vi "Find Rounded Error.vi"(1 "Camera Angle":dbl=35.25, 2 "Camera Axis Position":dbl) -> (0 "Rounded Error":dbl)   [LabVIEW 2012]
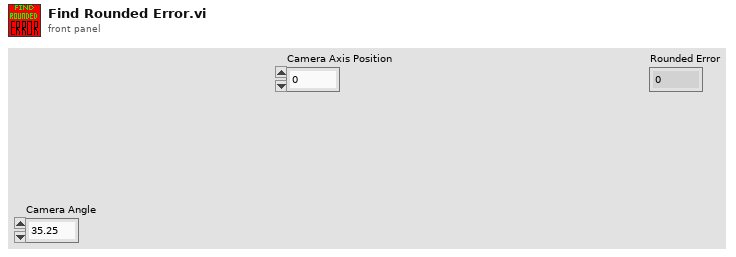
[diagram p1: front panel]
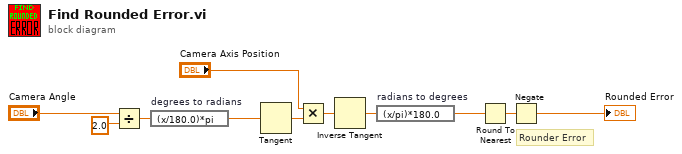
[diagram p0: block diagram]
diagram:
  # "Rounder Error"
  n1 = Divide(x="Camera Angle", y=2.0) -> (x/y=w4:dbl)
  n2 = expression code="(x/180.0)*pi" "degrees to radians"(w4) -> (w7:dbl)
  n3 = Tangent(1:w7) -> (0:w10:dbl)
  n4 = Multiply(x="Camera Axis Position", y=w10) -> (x*y=w8:dbl)
  n5 = Inverse Tangent(1:w8) -> (0:w9:dbl)
  n6 = expression code="(x/pi)*180.0" "radians to degrees"(w9) -> (w6:dbl)
  n7 = Round To Nearest(number=w6) -> (nearest integer value=w3:dbl)
  n8 = Negate(x=w3) -> (-x=→"Rounded Error":dbl)
